vi "Strip Commas and Whitespace.vi"(8 "error in (no error)":errorcluster, 11 "String to Strip":string) -> (0 "error out":errorcluster, 3 "Clean String":string)   [LabVIEW 2023, in "HAF.lvlib"]
uses:
  HAF.lvlib
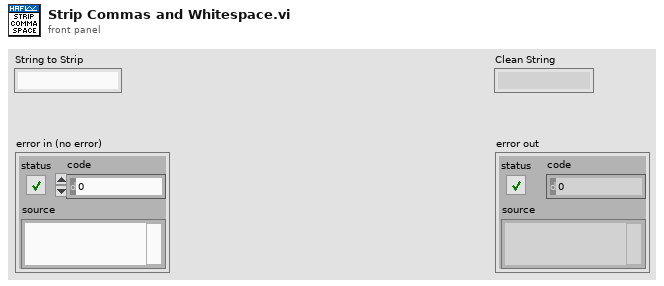
[diagram p1: front panel]
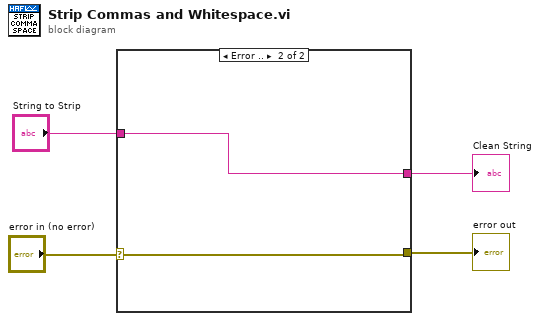
[diagram p0: block diagram]
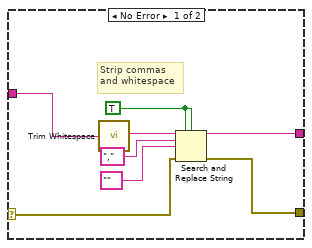
[diagram p2: hidden frame]
diagram:
  n1 = case shown="Error .." "error in (no error)" {
    selector: "error in (no error)" -> [w7 w13]
    tunnel: "String to Strip" -> [w8 w14]
    tunnel: [w6 w14] -> w2
    tunnel: [w5 w13] -> w1
    frame No Error {
      w9 = TRUE
      # "Strip commas\nand whitespace"
      n2 = call <vilib>:"Trim Whitespace.vi"("string"=w8) -> ("trimmed string"=w12:string)  [unwired: 1 in]
      n3 = Search and Replace String(replace all?=w9, case sensitive?=w9, input string=w12, search string=",", replace string="" ("replace string (\"\")"), error in=w7) -> (result string=w6:string, error out=w5:errorcluster)  [unwired: 2 in, 2 out]
    }
    frame Error {
    }
  }
  "Clean String" <- w2
  "error out" <- w1
